vi "checkIfControlInOldLibrary.vi"(8 "error in (no error)":errorcluster, 10 "Ctl Refnum":refnum<vi>, 11 "Dependency in":refnum<class "Dependency.lvclass">) -> (0 "error out":errorcluster, 1 "CtrlPath":path, 2 "isMemberOfOldLibrary":bool, 3 "Dependency out":refnum<class "Dependency.lvclass">)   [LabVIEW 2016, in "Dependency.lvclass"]
uses:
  Dependency.lvclass
  Dependency.lvclass/Dependency.ctl
  Search/Search.lvclass/Search.ctl
  Search/Search.lvclass
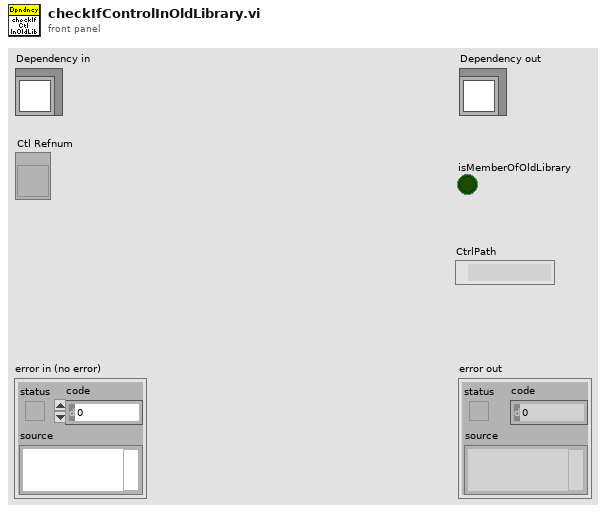
[diagram p1: front panel]
types:
  T1 = cluster{"OldLibrary":string, "NewLibrary":string}
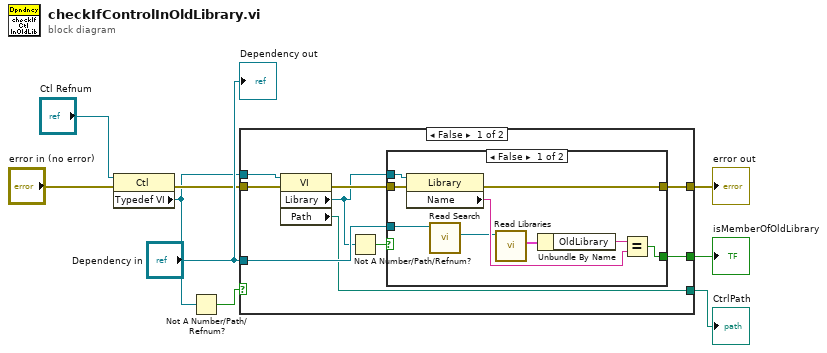
[diagram p0: block diagram]
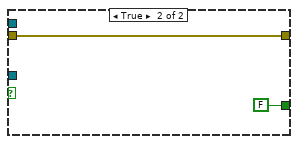
[diagram p2: hidden frame]
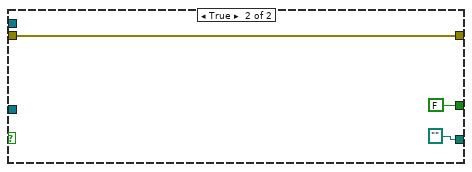
[diagram p3: hidden frame]
diagram:
  n1 = property class="Ctl"(reference="Ctl Refnum", error in="error in (no error)") -> (error out=w5:errorcluster, "Typedef VI"=w3:refnum<vi>)  [unwired: 1 out]
  n2 = Not A Number/Path/Refnum?(number/path/refnum=w3) -> (NaN/Path/Refnum?=w2:bool)
  n3 = case shown="False" w2 {
    tunnel: "Dependency in" -> [w18 _]
    tunnel: [w17 FALSE] -> w8
    tunnel: w5 -> [w16 w31]
    tunnel: [w14 w31] -> w4
    tunnel: w3 -> [w11 _]
    tunnel: [w10 path ""] -> w1
    frame False {
      n4 = property class="VI"(reference=w11, error in=w16) -> (error out=w15:errorcluster, "Library"=w13:refnum<vi>, "Path"=w10:path)  [unwired: 1 out]
      n5 = Not A Number/Path/Refnum?(number/path/refnum=w13) -> (NaN/Path/Refnum?=w12:bool)
      n6 = case shown="False" w12 {
        tunnel: w18 -> [w21 _]
        tunnel: [w25 FALSE] -> w17
        tunnel: w15 -> [w24 w28]
        tunnel: [w23 w28] -> w14
        tunnel: w13 -> [w22 _]
        frame False {
          n7 = property class="Library"(reference=w22, error in=w24) -> (error out=w23:errorcluster, "Name"=w26:string)  [unwired: 1 out]
          n8 = call "Read Search.vi"("Dependency in"=w21) -> ("Search"=w20:refnum<class "Search.lvclass">)  [unwired: 9 in, 1 out]
          n9 = call "Read Libraries.vi"("ProjectItem in"=w20) -> ("Libraries"=w19:T1)  [unwired: 9 in, 1 out]
          n10 = Unbundle By Name(w19) -> ("OldLibrary"=w27:string)
          n11 = Equal?(x=w27, y=w26) -> (x = y?=w25:bool)
        }
        frame True {
        }
      }
    }
    frame True {
    }
  }
  "error out" <- w4
  "isMemberOfOldLibrary" <- w8
  "CtrlPath" <- w1
  "Dependency out" <- "Dependency in"
